vi "path_plan.vi"(4 "Node2":string="C400D1", 5 "z":dbl=420.0, 6 "y":dbl=7988.0, 7 "x":dbl=8250.0) -> (0 "Path坐标数组":dbl[][](array[numeric]), 1 "Dis 2":dbl, 2 "Area 3":string[](array[string]), 3 "Path 2":string[](array[string]))   [LabVIEW 2014]
uses:
  <vilib>/Utility/importsl/GetValueByPointer/datatype.ctl
  <vilib>/Utility/importsl/GetValueByPointer/GetValueByPointer.xnode
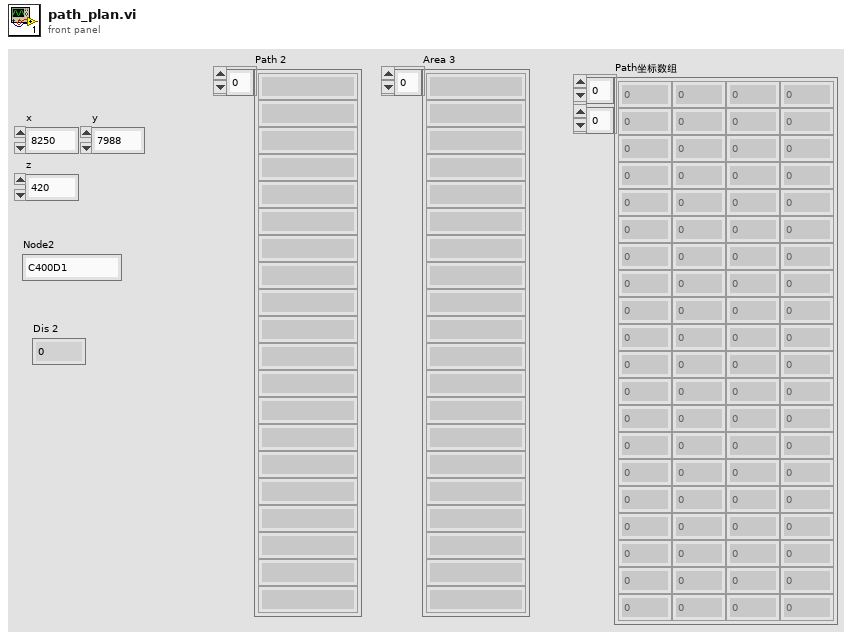
[diagram p1: front panel]
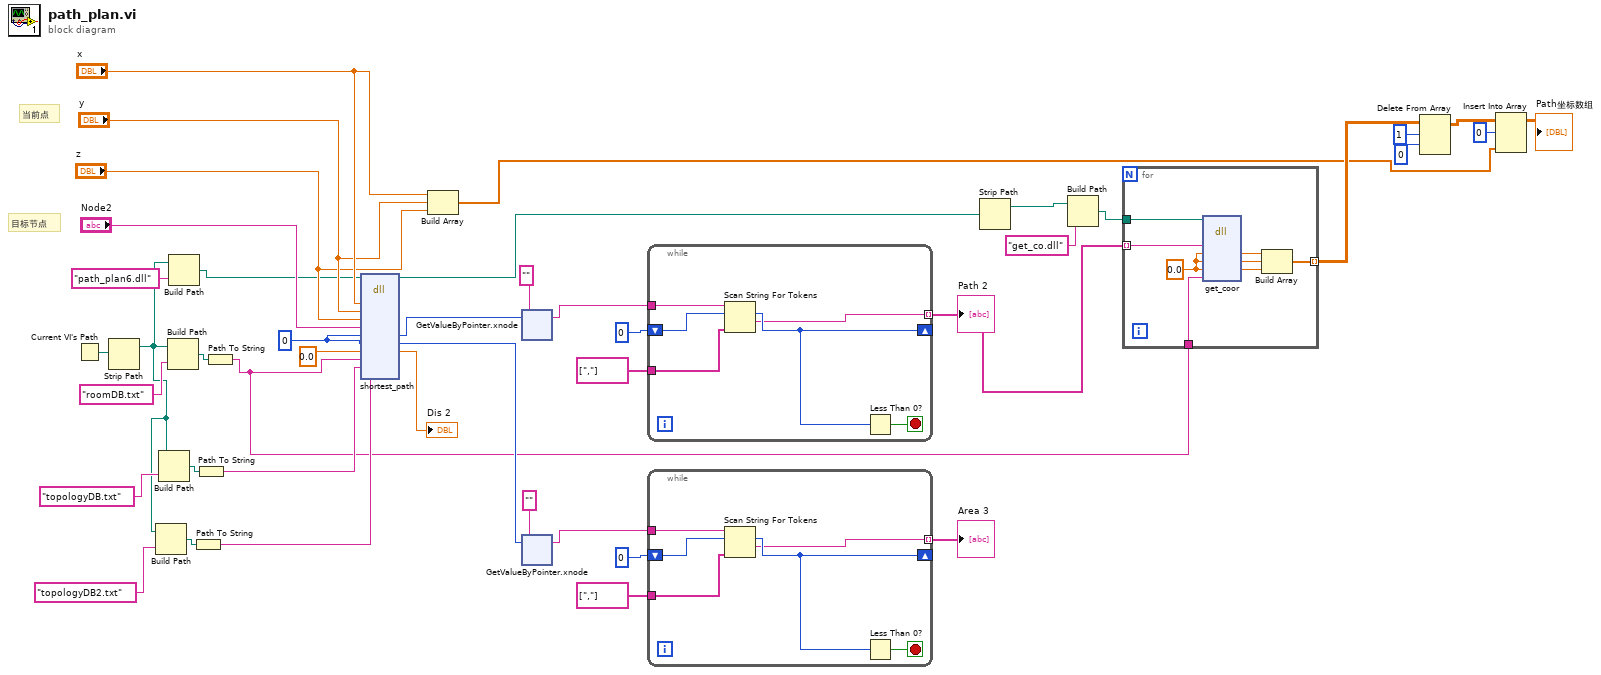
[diagram p0: block diagram]
diagram:
  w31 = 0 ("Path")
  # "目标节点"
  # "当前点"
  n1 = Current VI's Path() -> (path=w17:path)
  n2 = Strip Path(path=w17) -> (stripped path=w7:path)  [unwired: 1 out]
  n3 = Build Path(base path=w7, name or relative path="topologyDB2.txt" ("roomDB")) -> (appended path=w13:path)
  n4 = Build Path(base path=w7, name or relative path="topologyDB.txt" ("roomDB")) -> (appended path=w14:path)
  n5 = Build Path(base path=w7, name or relative path="roomDB.txt" ("roomDB")) -> (appended path=w16:path)
  n6 = Build Path(base path=w7, name or relative path="path_plan6.dll" ("名称或相对路径")) -> (appended path=w5:path)
  n7 = Path To String(path=w13) -> (string=w9:string)
  n8 = Path To String(path=w14) -> (string=w10:string)
  n9 = Path To String(path=w16) -> (string=w8:string)
  n10 = dll-call lib="E:/labview/1511/zsControlSystem2.0/FromOtherProject/FromLXY/speech/path_plan6.dll" fn="shortest_path"(path in=w5, "X"="x", "Y"="y", "Z"="z", "Node2"="Node2", "Path"=w31, "Area"=w31, "Dis"=0.0, "roomDB"=w8, "topologyDB"=w10, "topologyDB2"=w9) -> (path out=w4:path, "Path"=w34:i32, "Area"=w32:i32, "Dis"=→"Dis 2":dbl)  [unwired: 10 in, 1 out]
  n11 = Build Array("x", "y", "z") -> (w19:dbl[])
  n12 = xnode "GetValueByPointer.xnode"("Pointer"=w34, "InputType"="") -> ("Output"=w40:string)  [unwired: 2 in, 1 out]
  n13 = xnode "GetValueByPointer.xnode"("Pointer"=w32, "InputType"="") -> ("Output"=w35:string)  [unwired: 2 in, 1 out]
  n14 = while {
    shift-right: [w47] -> _
    shift-left: 0 -> [w49]
    tunnel: [w46] -> w29 mode=indexing
    tunnel: string[] [","] ("分隔符(\\s,\\t,\\r,\\n)") -> [w45]
    tunnel: w40 -> [w44]
    stop <- w48 stop-if-true
    n15 = Scan String For Tokens(6:w45, 8:w49, 9:w44) -> (1:w46:string, 2:w47:i32)  [unwired: 3 in, 2 out]
    n16 = Less Than 0?(x=w47) -> (x < 0?=w48:bool)
  }
  "Path 2" <- w29
  n17 = while {
    shift-right: [w53] -> _
    shift-left: 0 -> [w55]
    tunnel: [w52] -> w37 mode=indexing
    tunnel: string[] [","] ("分隔符(\\s,\\t,\\r,\\n)") -> [w51]
    tunnel: w35 -> [w50]
    stop <- w54 stop-if-true
    n18 = Scan String For Tokens(6:w51, 8:w55, 9:w50) -> (1:w52:string, 2:w53:i32)  [unwired: 3 in, 2 out]
    n19 = Less Than 0?(x=w53) -> (x < 0?=w54:bool)
  }
  "Area 3" <- w37
  n20 = Strip Path(path=w4) -> (stripped path=w3:path)  [unwired: 1 out]
  n21 = Build Path(base path=w3, name or relative path="get_co.dll" ("名称或相对路径")) -> (appended path=w1:path)
  n22 = for {
    tunnel: w29 -> [w59] mode=indexing
    tunnel: [w58] -> w24 mode=indexing
    tunnel: w8 -> [w57]
    tunnel: w1 -> [w56]
    w63 = 0.0 ("参数2")
    n23 = dll-call lib="E:/labview/1511/zsControlSystem2.0/FromOtherProject/FromLXY/speech/get_co.dll" fn="get_coor"(path in=w56, "Node"=w59, "X"=w63, "Y"=w63, "Z"=w63, "Room"=w57) -> ("X"=w62:dbl, "Y"=w61:dbl, "Z"=w60:dbl)  [unwired: 5 in, 2 out]
    n24 = Build Array(w62, w61, w60) -> (w58:dbl[])
  }
  n25 = Delete From Array(array=w24, length=1 ("长度"), index (row)=0 ("索引 (行)")) -> (array with subset deleted=w21:dbl[][])  [unwired: 1 in, 1 out]
  n26 = Insert Into Array(array=w21, index (row)=0 ("索引 (行)"), new element=w19) -> (→"Path坐标数组":dbl[][])  [unwired: 1 in]
